vi "Write to Log.vi"(8 "error in (no error)":errorcluster, 11 "Log In":string) -> (0 "error out":errorcluster)   [LabVIEW 2012]
panel:
  out "Exe time":u32
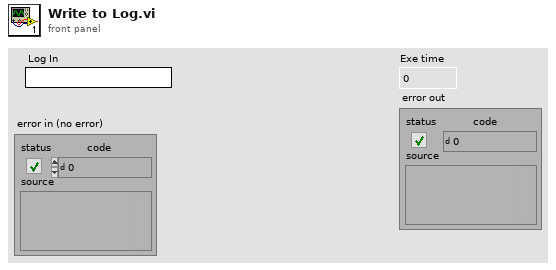
[diagram p1: front panel]
types:
  T1 = enum16{"open", "replace", "create", "open or create", "replace or create", "replace or create with confirmation"}
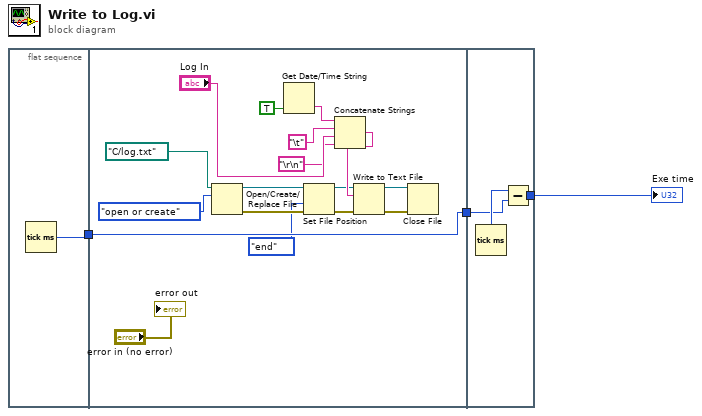
[diagram p0: block diagram]
diagram:
  n1 = flat-sequence {
    tunnel: [w4] -> w2
    tunnel: [w12] -> w3
    tunnel: w2 -> [w12]
    tunnel: w3 -> [w23]
    tunnel: [w22] -> w1
    frame #0 {
      n2 = Tick Count (ms)() -> (millisecond timer value=w4:u32)
    }
    frame #1 {
      n3 = Open/Create/Replace File(file path (use dialog)=path "C:/log.txt", operation (0:open)=T1."open or create") -> (refnum out=w7:refnum<file>, error out=w8:errorcluster)  [unwired: 4 in, 1 out]
      n4 = Get Date/Time String(want seconds? (F)=TRUE) -> (time string=w18:string)  [unwired: 2 in, 1 out]
      n5 = Set File Position(refnum=w7, from (0:start)=enum16{"start", "end", "current"}."end", error in=w8) -> (refnum out=w10:refnum<file>, error out=w9:errorcluster)  [unwired: 1 in]
      n6 = Concatenate Strings(w18, "\t", "Log In", "\r\n") -> (w15:string)
      n7 = Write to Text File(file (use dialog)=w10, text=w15, error in=w9) -> (refnum out=w14:refnum<file>, error out=w13:errorcluster)  [unwired: 1 in, 1 out]
      n8 = Close File(refnum=w14, error in=w13) -> ()  [unwired: 2 out]
      "error out" <- "error in (no error)"
    }
    frame #2 {
      n9 = Tick Count (ms)() -> (millisecond timer value=w24:u32)
      n10 = Subtract(x=w24, y=w23) -> (x-y=w22:u32)
    }
  }
  "Exe time" <- w1
